vi "MAIN_Update_ASI_stage_position.vi"(3 "error in":errorcluster, 5 "XY positions":dbl[][](array[numeric])) -> (0 "error out":errorcluster, 1 "XY positions OUT":dbl[][](array[numeric]), 2 "XYZ":cluster{"x(um)":dbl, "y(um)":dbl, "z(um)":dbl} {"x(um)" format="%#.1f"; "y(um)" format="%#.1f"; "z(um)" format="%#.1f"})   [LabVIEW 2015]
uses:
  GLOBAL/Global_ASI_stage.vi
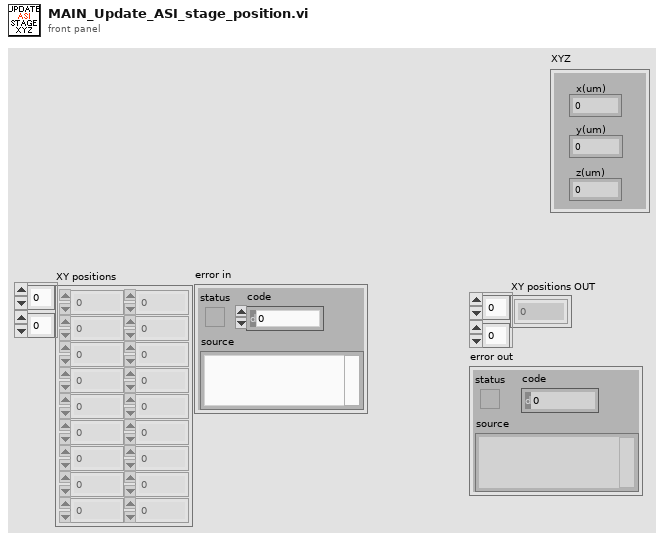
[diagram p1: front panel]
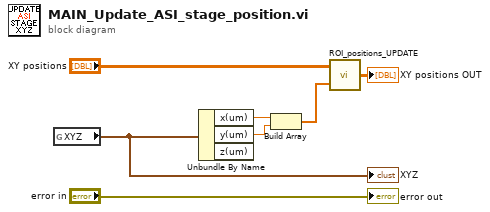
[diagram p0: block diagram]
diagram:
  n1 = global read "Global_ASI_stage.vi" "XYZ"() -> (w1:cluster{"x(um)":dbl, "y(um)":dbl, "z(um)":dbl})
  "XYZ" <- w1
  n2 = Unbundle By Name(w1) -> ("x(um)"=w3:dbl, "y(um)"=w2:dbl)  [unwired: 1 out]
  n3 = Build Array(w3, w2) -> (w7:dbl[])
  n4 = call "ROI_positions_UPDATE.vi"("XY new position"=w7, "XY positions IN"="XY positions") -> ("XY positions OUT"=→"XY positions OUT":dbl[][])
  "error out" <- "error in"
